vi "Monitor_Setting.vi"(8 "Error in":errorcluster) -> (0 "error out 2":errorcluster)   [LabVIEW 2017]
uses:
  System.Windows.Forms
  System.Drawing
  <vilib>/Utility/config.llb/NI_LVConfig.lvlib
  <vilib>/Utility/config.llb/Read Key (Boolean).vi
panel:
  in  "Printer IP 3":string
  in  "Printer IP 2":string
  in  "Printer IP 1":string
  in  "Scanner IP 3":string
  in  "Scanner IP 2":string
  in  "Scanner IP 1":string
  in  "Save Setting":bool
  in  "Monitor 3":u16
  in  "Monitor 2":u16
  in  "Monitor Primary 1":u16
  in  "screen number":u16=1
  out "Current Monitor Status":bool
  out "Current Monitor Number":u16
  in  "Refresh Monitors":bool
  out "Monitor H and W":i32[][](array[numeric])
  out "Display Names":string[](array[string])
  out "Primary Monitor\nMethod 2":i32
  in  "Close":bool
  out "error out":errorcluster
  out "Machine Name":string
  # "Resolution: 1920 x 1080 pixels"
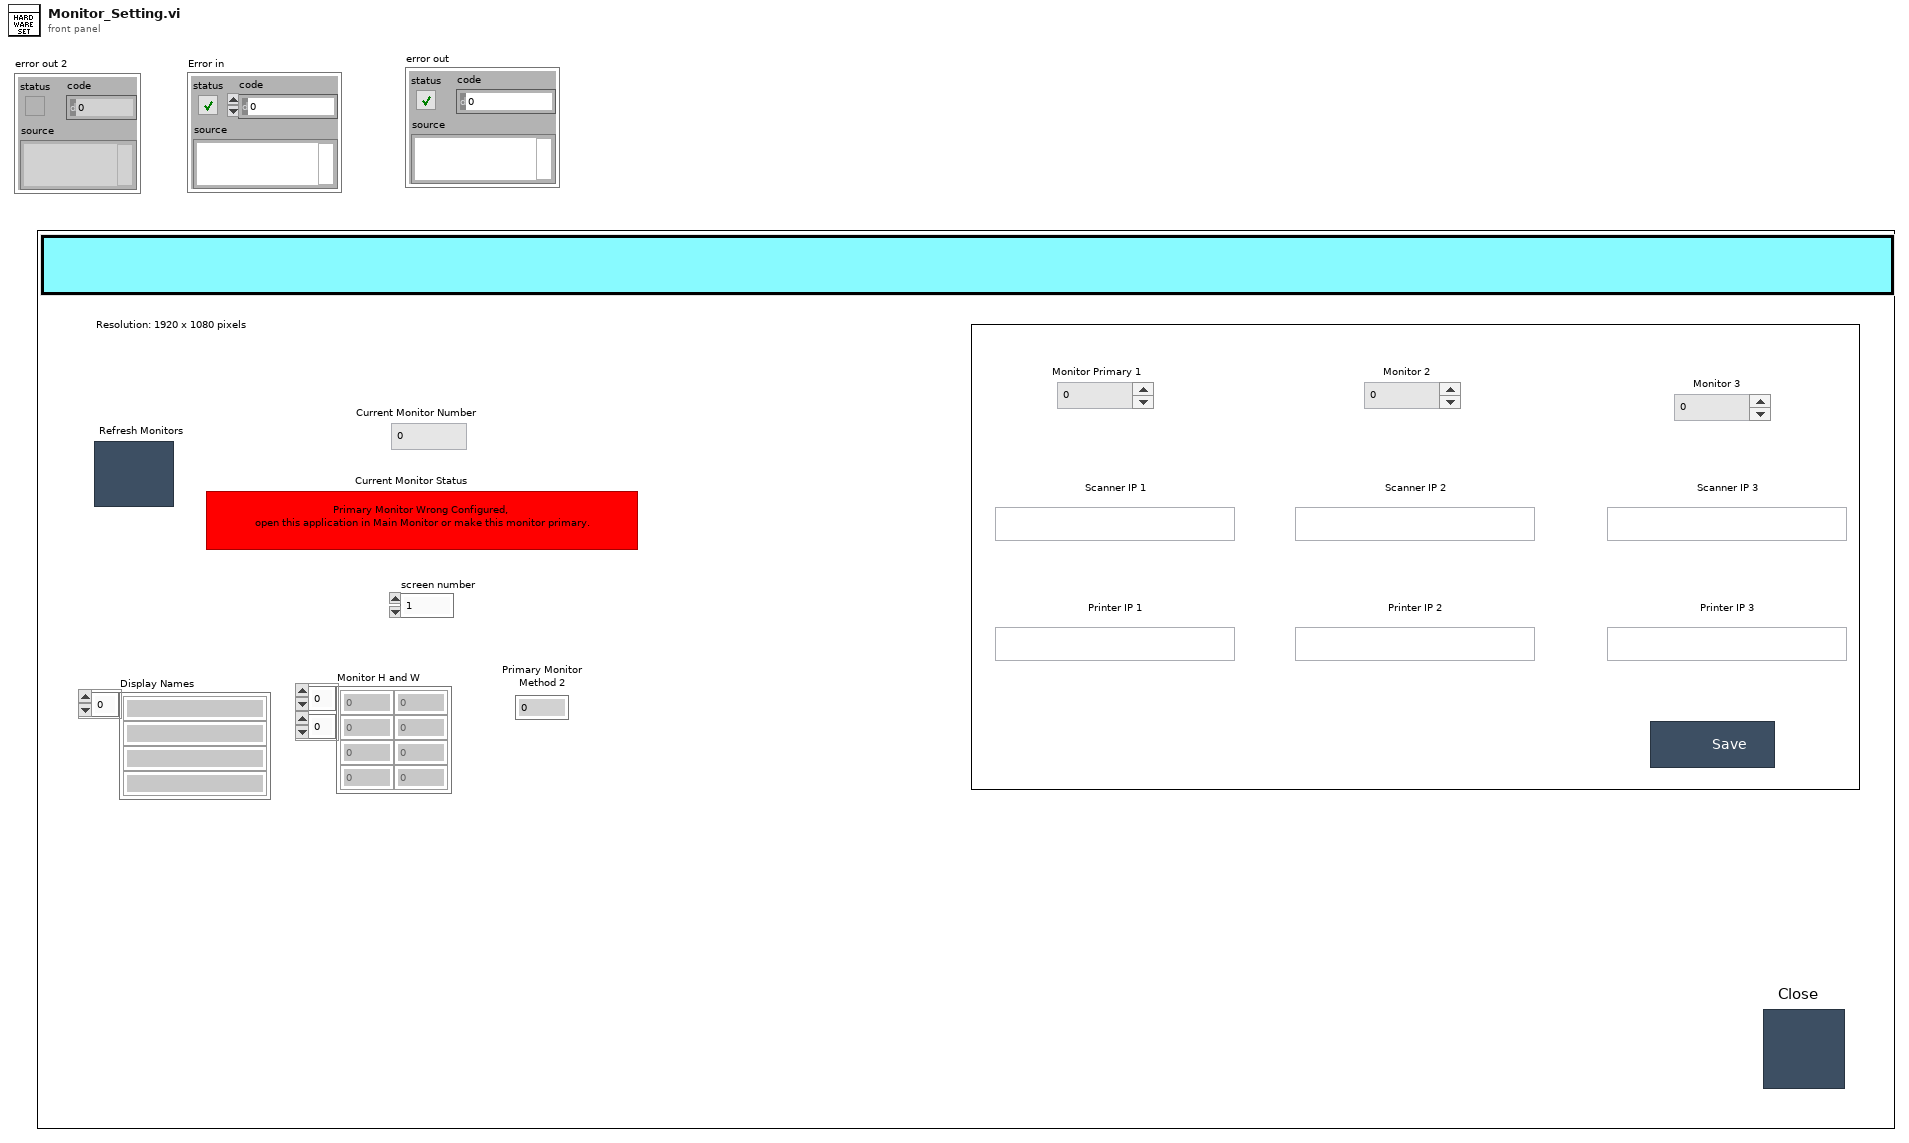
[diagram p1: front panel]
types:
  T1 = cluster{"Monitor Primary 1":u16, "Monitor 2":u16, "Monitor 3":u16, "Scanner IP 1":string, "Scanner IP 2":string, "Scanner IP 3":string, "Printer IP 1":string, "Printer IP 2":string, "Printer IP 3":string}
  T2 = enum32{"invalid app kind", "Development System", "Run Time System", "Student Edition", "Embedded LabVIEW", "Evaluation", "Custom"}
  T3 = typedef "NI_LVConfig.lvlib/Config Data RefNum.ctl" = refnum<k1>
  T4 = enum32{"Invalid", "Standard", "Closed", "Hidden", "Minimized", "Maximized"}
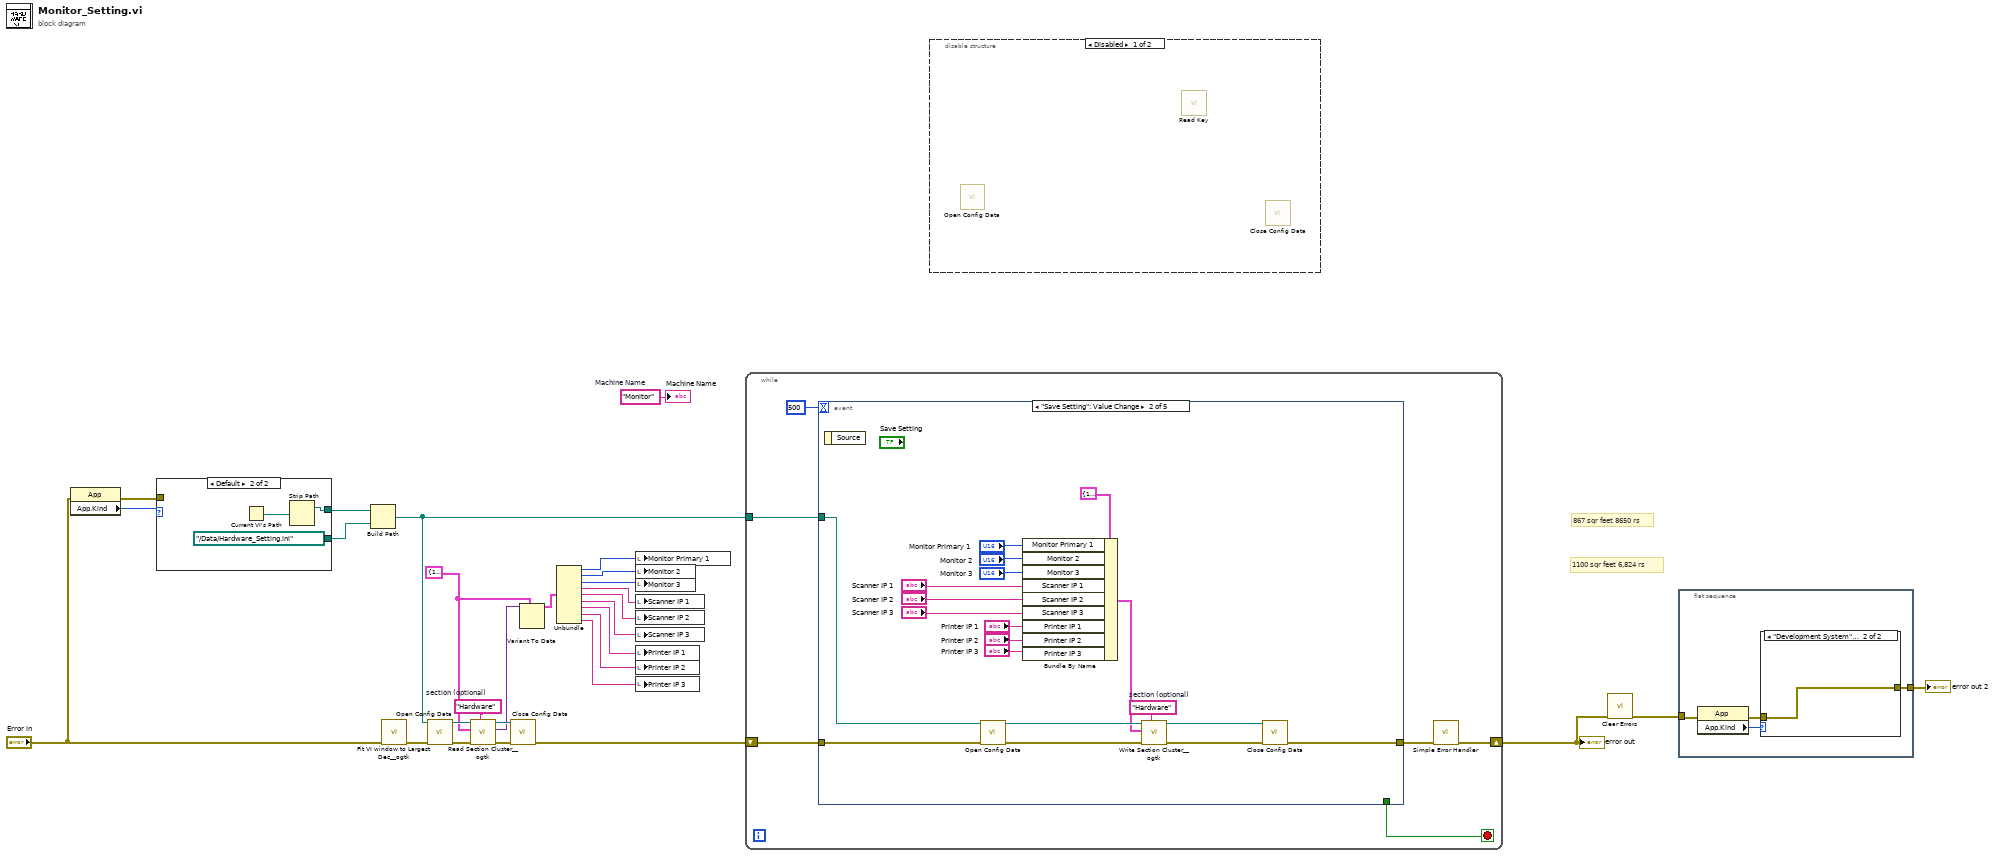
[diagram p0: block diagram]
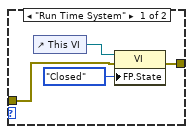
[diagram p2: hidden frame]
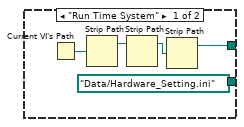
[diagram p4: hidden frame]
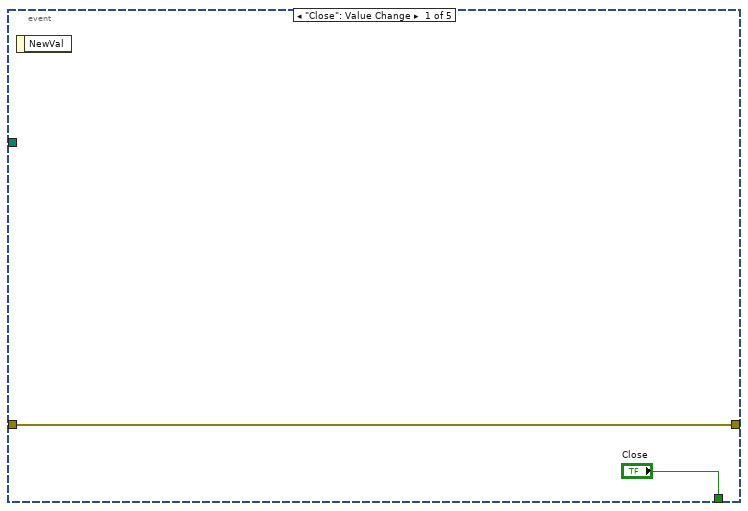
[diagram p5: hidden frame]
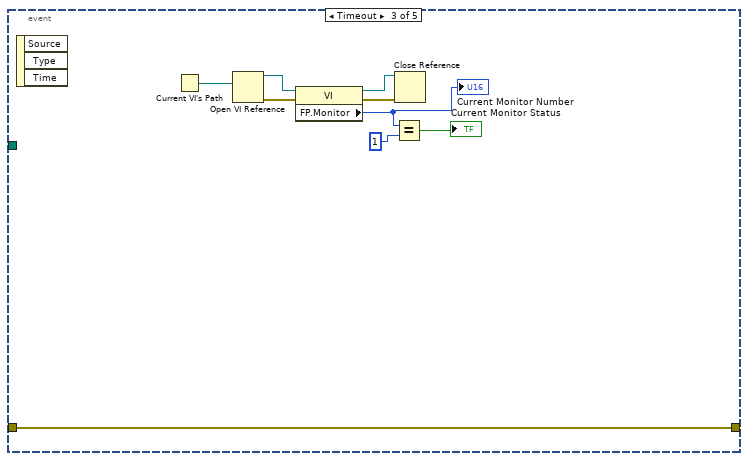
[diagram p6: hidden frame]
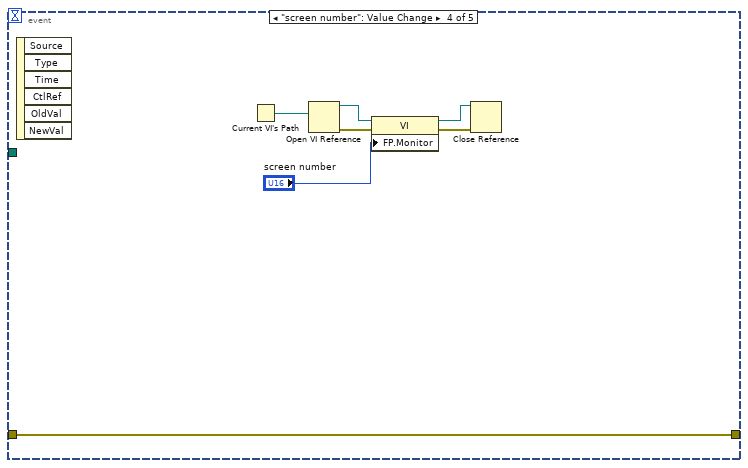
[diagram p7: hidden frame]
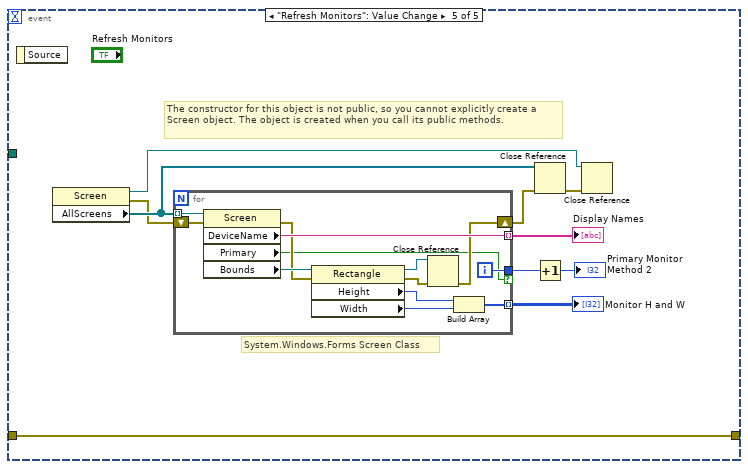
[diagram p8: hidden frame]
diagram:
  w7 = T1 {"Monitor Primary 1"=1, "Monitor 2"=2, "Monitor 3"=3, "Scanner IP 1"="", "Scanner IP 2"="", "Scanner IP 3"="", "Printer IP 1"="", "Printer IP 2"="", "Printer IP 3"=""}
  w15 = "Hardware"  # section (optional)
  w29 = "Monitor"  # Machine Name
  # "1100 sqr feet 6,824 rs"
  # "867 sqr feet 8650 rs"
  n1 = property class="App"(error in="Error in") -> (error out=w26:errorcluster, "App.Kind"=w28:T2)  [unwired: 1 in, 1 out]
  n2 = case shown="Default" w28 {
    tunnel: [path "Data/Hardware_Setting.ini" ("path") path "../Data/Hardware_Setting.ini" ("path")] -> w27
    tunnel: [w30 w35] -> w25
    tunnel: w26 -> [_ _]
    frame "Run Time System" {
      n3 = Current VI's Path() -> (path=w33:path)
      n4 = Strip Path(path=w33) -> (stripped path=w32:path)  [unwired: 1 out]
      n5 = Strip Path(path=w32) -> (stripped path=w31:path)  [unwired: 1 out]
      n6 = Strip Path(path=w31) -> (stripped path=w30:path)  [unwired: 1 out]
    }
    frame Default {
      n7 = Current VI's Path() -> (path=w36:path)
      n8 = Strip Path(path=w36) -> (stripped path=w35:path)  [unwired: 1 out]
    }
  }
  n9 = Build Path(base path=w25, name or relative path=w27) -> (appended path=w22:path)
  n10 = call <userlib>:"Fit VI window to Largest Dec__ogtk.vi"("error in (no error)"="Error in") -> ("error out"=w18:errorcluster)  [unwired: 5 in, 1 out]
  n11 = call <vilib>:"Open Config Data.vi"("error in (no error)"=w18, "configuration file path"=w22) -> ("error out"=w17:errorcluster, "refnum"=w13:T3)  [unwired: 7 in, 1 out]
  n12 = call <userlib>:"Read Section Cluster__ogtk.vi"("section (optional)"=w15, "error in (no error)"=w17, "Section Formatted Cluster Type"=w7, "refnum"=w13) -> ("error out"=w16:errorcluster, "Section Formatted Cluster"=w12:variant, "dup refnum"=w14:T3)  [unwired: 3 in, 2 out]
  n13 = call <vilib>:"Close Config Data.vi"("error in (no error)"=w16, "refnum"=w14) -> ("error out"=w23:errorcluster)  [unwired: 8 in, 1 out]
  n14 = Variant To Data(type=w7, Variant=w12) -> (data=w11:T1)  [unwired: 1 in, 1 out]
  n15 = Unbundle(w11) -> ("Monitor Primary 1"=w10:u16, "Monitor 2"=w9:u16, "Monitor 3"=w8:u16, "Scanner IP 1"=w6:string, "Scanner IP 2"=w5:string, "Scanner IP 3"=w4:string, "Printer IP 1"=w3:string, "Printer IP 2"=w2:string, "Printer IP 3"=w1:string)
  n16 = local write "Monitor Primary 1"(w10) -> ()
  n17 = local write "Monitor 2"(w9) -> ()
  n18 = local write "Monitor 3"(w8) -> ()
  n19 = local write "Scanner IP 1"(w6) -> ()
  n20 = local write "Scanner IP 2"(w5) -> ()
  n21 = local write "Scanner IP 3"(w4) -> ()
  n22 = local write "Printer IP 1"(w3) -> ()
  n23 = local write "Printer IP 2"(w2) -> ()
  n24 = local write "Printer IP 3"(w1) -> ()
  n25 = while {
    shift-right: [w38] -> w20
    shift-left: w23 -> [w41]
    tunnel: w22 -> [w39]
    stop <- w43 stop-if-true
    n26 = event shown="[1] \"Save Setting\": Value Change" {
      selector: _ -> [_ _ _ _ _]
      dyn-events: _ -> [_ _ _ _ _]
      timeout: 500 -> [_ _ _ _ _]
      tunnel: ["Close" _ _ _ _] -> w43
      tunnel: [w44 w61 w68 w74 w81] -> w42
      tunnel: w41 -> [w44 w62 w68 w74 w81]
      tunnel: w39 -> [_ w63 _ _ _]
      event "Close": Value Change {
        n27 = event-data() -> ()  [unwired: 1 in, 1 out]
      }
      event "Save Setting": Value Change {
        w59 = "Hardware"  # section (optional)
        n28 = event-data() -> ()  [unwired: 1 in, 1 out]
        n29 = call <vilib>:"Open Config Data.vi"("error in (no error)"=w62, "configuration file path"=w63) -> ("error out"=w58:errorcluster, "refnum"=w64:T3)  [unwired: 7 in, 1 out]
        n30 = Bundle By Name(cluster=T1 {"Monitor Primary 1"=1, "Monitor 2"=2, "Monitor 3"=3, "Scanner IP 1"="", "Scanner IP 2"="", "Scanner IP 3"="", "Printer IP 1"="", "Printer IP 2"="", "Printer IP 3"=""}, "Monitor Primary 1"="Monitor Primary 1", "Monitor 2"="Monitor 2", "Monitor 3"="Monitor 3", "Scanner IP 1"="Scanner IP 1", "Scanner IP 2"="Scanner IP 2", "Scanner IP 3"="Scanner IP 3", "Printer IP 1"="Printer IP 1", "Printer IP 2"="Printer IP 2", "Printer IP 3"="Printer IP 3") -> (w53:T1)
        n31 = call <userlib>:"Write Section Cluster__ogtk.vi"("section (optional)"=w59, "error in (no error)"=w58, "Section Formatted Cluster"=w53, "refnum"=w64) -> ("error out"=w57:errorcluster, "dup refnum"=w60:T3)  [unwired: 6 in]
        n32 = call <vilib>:"Close Config Data.vi"("error in (no error)"=w57, "refnum"=w60) -> ("error out"=w61:errorcluster)  [unwired: 8 in, 1 out]
      }
      event Timeout {
        n33 = event-data() -> ()  [unwired: 1 in, 3 out]
        n34 = Current VI's Path() -> (path=w73:path)
        n35 = Open VI Reference(vi path=w73) -> (vi reference=w69:refnum<vi>, error out=w70:errorcluster)  [unwired: 5 in]
        n36 = property class="VI"(reference=w69, error in=w70) -> (reference out=w72:refnum<vi>, error out=w71:errorcluster, "FP.Monitor"=w65:u16)
        "Current Monitor Number" <- w65
        n37 = Equal?(x=w65, y=u16 1) -> (x = y?=→"Current Monitor Status":bool)
        n38 = Close Reference(reference=w72, error in (no error)=w71) -> ()  [unwired: 1 out]
      }
      event "screen number": Value Change {
        n39 = event-data() -> ()  [unwired: 1 in, 6 out]
        n40 = Current VI's Path() -> (path=w79:path)
        n41 = Open VI Reference(vi path=w79) -> (vi reference=w75:refnum<vi>, error out=w76:errorcluster)  [unwired: 5 in]
        n42 = property class="VI"(reference=w75, error in=w76, "FP.Monitor"="screen number") -> (reference out=w78:refnum<vi>, error out=w77:errorcluster)
        n43 = Close Reference(reference=w78, error in (no error)=w77) -> ()  [unwired: 1 out]
      }
      event "Refresh Monitors": Value Change {
        # "System.Windows.Forms Screen Class"
        # "The constructor for this object is not public, so you cannot explicitly create a Screen object. The object is created when you call its public methods."
        n44 = event-data() -> ()  [unwired: 1 in, 1 out]
        n45 = property class="Screen"() -> (reference out=w87:refnum<k24>, error out=w83:errorcluster, "AllScreens"=w85:refnum<k24>[])  [unwired: 2 in]
        n46 = for {
          tunnel: w85 -> [w103] mode=indexing
          tunnel: [w102] -> w82 mode=indexing
          shift-right: [w96] -> w84
          shift-left: w83 -> [w100]
          tunnel: [w95] -> w88 if=w94
          tunnel: [w91] -> w89 mode=indexing
          i -> [w95]
          n47 = property class="Screen"(reference=w103, error in=w100) -> (error out=w97:errorcluster, "DeviceName"=w102:string, "Primary"=w94:bool, "Bounds"=w101:refnum<k24>)  [unwired: 1 out]
          n48 = property class="Rectangle"(reference=w101, error in=w97) -> (reference out=w98:refnum<k24>, error out=w99:errorcluster, "Height"=w93:i32, "Width"=w92:i32)
          n49 = Close Reference(reference=w98, error in (no error)=w99) -> (error out=w96:errorcluster)
          n50 = Build Array(w93, w92) -> (w91:i32[])
        }
        "Display Names" <- w82
        "Monitor H and W" <- w89
        n51 = Close Reference(reference=w85, error in (no error)=w84) -> (error out=w86:errorcluster)
        n52 = Increment(x=w88) -> (x+1=→"Primary Monitor\nMethod 2":i32)
        n53 = Close Reference(reference=w87, error in (no error)=w86) -> ()  [unwired: 1 out]
      }
    }
    n54 = call <vilib>:"Simple Error Handler.vi"("error in (no error)"=w42) -> ("error out"=w38:errorcluster)  [unwired: 4 in, 4 out]
  }
  "error out" <- w20
  n55 = disable-structure shown="Disabled" {
    frame Disabled {
      n56 = call <vilib>:"Open Config Data.vi"() -> ()  [unwired: 9 in, 3 out]
      n57 = call-poly <vilib>:"Read Key.vi"() -> ()  [unwired: 8 in, 4 out]
      n58 = call <vilib>:"Close Config Data.vi"() -> ()  [unwired: 10 in, 2 out]
    }
    frame Enabled {
    }
  }
  n59 = call <vilib>:"Clear Errors.vi"("error in (no error)"=w20) -> ("error out"=w19:errorcluster)  [unwired: 5 in, 1 out]
  n60 = flat-sequence {
    tunnel: [w105] -> w21
    tunnel: w19 -> [w104]
    frame #0 {
      n61 = property class="App"(error in=w104) -> (error out=w106:errorcluster, "App.Kind"=w107:T2)  [unwired: 1 in, 1 out]
      n62 = case shown="\"Development System\", Default" w107 {
        tunnel: w106 -> [w109 w112]
        tunnel: [w108 w112] -> w105
        frame "Run Time System" {
          n63 = control-ref of="This VI"() -> (w111:refnum<vi>)
          n64 = property class="VI"(reference=w111, error in=w109, "FP.State"=T4."Closed" ("Front Panel Window:State")) -> (error out=w108:errorcluster)  [unwired: 1 out]
        }
        frame "Development System", Default {
        }
      }
    }
  }
  "Machine Name" <- w29
  "error out 2" <- w21
